vi "test Diff Configuration (Add Port).vi"(8 "error in":errorcluster, 11 "TestCase in":refnum<class "Refresh.lvclass">) -> (0 "error out":errorcluster, 3 "TestCase out":refnum<class "Refresh.lvclass">)   [LabVIEW 2020, in "Refresh.lvclass"]
uses:
  Refresh.lvclass
  System Explorer/Implementation/System Explorer/Refresh/MCL Row.ctl
  System Explorer/Implementation/System Explorer/Refresh/Change Type.ctl
  System Explorer/Implementation/System Explorer/Refresh/Symbols.ctl
  Shared/1553 Channel.ctl
  Shared/Address.ctl
  Shared/Message Definition.ctl
  Shared/Message Type.ctl
  Shared/Terminal Endpoint.ctl
  Shared/Parameter Definition.ctl
  <vilib>/addons/_JKI Toolkits/VI Tester/TestCase.llb/TestCase.lvclass
  System Explorer/Implementation/System Explorer/Refresh/Refresh.lvlib
  C:/Program Files (x86)/National Instruments/LabVIEW 2020/vi.lib/addons/_JKI Toolkits/VI Tester/TestCase.llb/TestCase.lvclass
panel:
  out "Multicolumn Listbox":i32(listbox)=-1
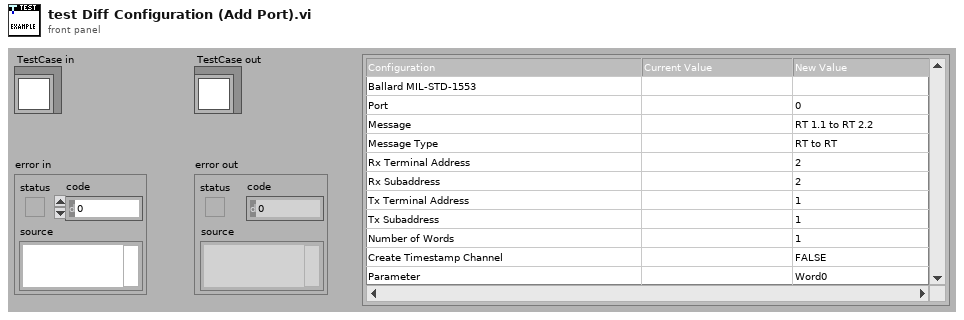
[diagram p1: front panel]
types:
  T1 = typedef "Message Definition.ctl" = cluster{"name":string, "message type":T2, "endpoint Tx":T3, "endpoint Rx":T3, "create timestamp channel":bool, "mode code":u16, "number of words":u16, "parameters":cluster{"name":string, "default value":dbl, "unit":string, "parameter definition":T5}[]}
  T2 = typedef "Message Type.ctl" = string
  T3 = typedef "Terminal Endpoint.ctl" = cluster{"terminal address":T4, "subaddress":T4}
  T4 = typedef "Address.ctl" = u16
  T5 = typedef "Parameter Definition.ctl" = cluster{"start index":i32, "size (bits)":i32, "encoding":enum16{"BNR", "BCD", "Discrete"}, "signed":bool, "multiplier":dbl, "offset":dbl}
  T6 = typedef "1553 Channel.ctl" = cluster{"HW channel":u16, "terminal addresses":T4[], "acyclic frame names":string[], "messages":T1[]}
  T7 = typedef "Ballard MIL-STD-1553 System Explorer.lvlib/Implementation.lvlib/Refresh.lvlib/MCL Row.ctl" = cluster{"change type":T8, "item symbol":T9, "item names":string[]}
  T8 = typedef "Ballard MIL-STD-1553 System Explorer.lvlib/Implementation.lvlib/Refresh.lvlib/Change Type.ctl" = enum16{"No change", "Modify", "Add", "Remove"}
  T9 = typedef "Ballard MIL-STD-1553 System Explorer.lvlib/Implementation.lvlib/Refresh.lvlib/Symbols.ctl" = enum16{"Blank", "MIL-STD-1553", "Port", "Remote Terminal", "Subaddress", "Bus Controller", "Acyclic Frame", "Mode Code", "Message", "Parameter", "Item"}
  T10 = typedef "imagedata.ctl" = cluster{"image type":i32, "image depth":i32, "image":u8[], "mask":u8[], "colors":u32[], "Rectangle":cluster{"left":i16, "top":i16, "right":i16, "bottom":i16}}
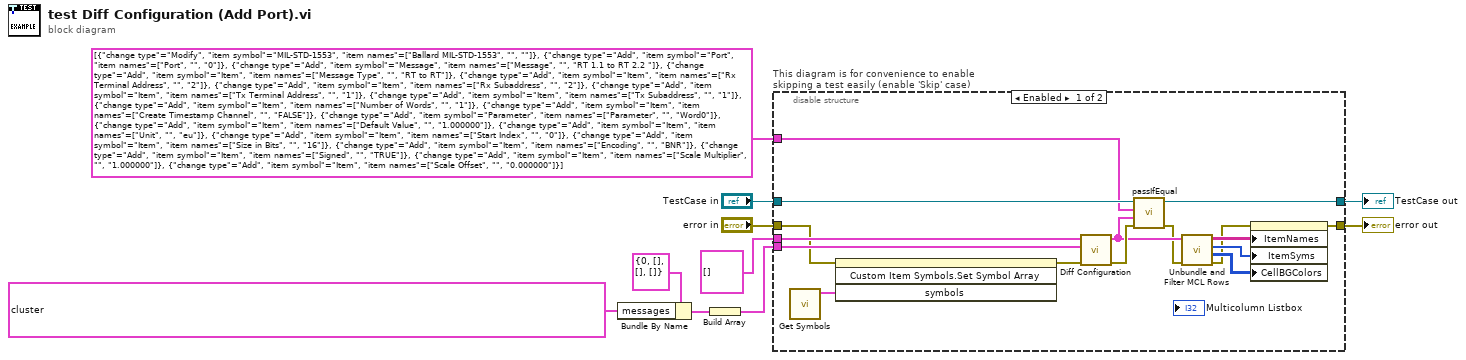
[diagram p0: block diagram]
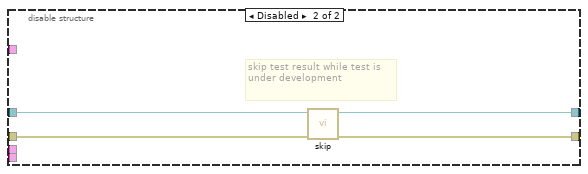
[diagram p2: hidden frame]
diagram:
  n1 = Bundle By Name(cluster=T6 {"HW channel"=0, "terminal addresses"=[], "acyclic frame names"=[], "messages"=[]} ("1553 channel"), "messages"=T1[] [{"name"="RT 1.1 to RT 2.2 ", "message type"="RT to RT", "endpoint Tx"={"terminal address"=1, "subaddress"=1}, "endpoint Rx"={"terminal address"=2, "subaddress"=2}, "create timestamp channel"=FALSE, "mode code"=0, "number of words"=1, "parameters"=[{"name"="Word0", "default value"=1.0, "unit"="eu", "parameter definition"={"start index"=0, "size (bits)"=16, "encoding"=enum."BNR", "signed"=TRUE, "multiplier"=1.0, "offset"=0.0}}]}]) -> (w1:T6)
  n2 = Build Array(w1) -> (w5:T6[])
  n3 = disable-structure "This diagram is for convenience to enable skipping a test easily (enable 'Skip' case)" shown="Enabled" {
    disable-tunnel: "TestCase in" -> [w26 w30]
    disable-tunnel: [w25 w28] -> w7
    disable-tunnel: [w14 w29] -> w9
    disable-tunnel: "error in" -> [w12 w27]
    disable-tunnel: T6[] [] -> [w24 _]
    disable-tunnel: w5 -> [w23 _]
    disable-tunnel: T7[] [{"change type"=enum."Modify", "item symbol"=enum."MIL-STD-1553", "item names"=["Ballard MIL-STD-1553", "", ""]}, {"change type"=enum."Add", "item symbol"=enum."Port", "item names"=["Port", "", "0"]}, {"change type"=enum."Add", "item symbol"=enum."Message", "item names"=["Message", "", "RT 1.1 to RT 2.2 "]}, {"change type"=enum."Add", "item symbol"=enum."Item", "item names"=["Message Type", "", "RT to RT"]}, {"change type"=enum."Add", "item symbol"=enum."Item", "item names"=["Rx Terminal Address", "", "2"]}, {"change type"=enum."Add", "item symbol"=enum."Item", "item names"=["Rx Subaddress", "", "2"]}, {"change type"=enum."Add", "item symbol"=enum."Item", "item names"=["Tx Terminal Address", "", "1"]}, {"change type"=enum."Add", "item symbol"=enum."Item", "item names"=["Tx Subaddress", "", "1"]}, {"change type"=enum."Add", "item symbol"=enum."Item", "item names"=["Number of Words", "", "1"]}, {"change type"=enum."Add", "item symbol"=enum."Item", "item names"=["Create Timestamp Channel", "", "FALSE"]}, {"change type"=enum."Add", "item symbol"=enum."Parameter", "item names"=["Parameter", "", "Word0"]}, {"change type"=enum."Add", "item symbol"=enum."Item", "item names"=["Default Value", "", "1.000000"]}, {"change type"=enum."Add", "item symbol"=enum."Item", "item names"=["Unit", "", "eu"]}, {"change type"=enum."Add", "item symbol"=enum."Item", "item names"=["Start Index", "", "0"]}, {"change type"=enum."Add", "item symbol"=enum."Item", "item names"=["Size in Bits", "", "16"]}, {"change type"=enum."Add", "item symbol"=enum."Item", "item names"=["Encoding", "", "BNR"]}, {"change type"=enum."Add", "item symbol"=enum."Item", "item names"=["Signed", "", "TRUE"]}, {"change type"=enum."Add", "item symbol"=enum."Item", "item names"=["Scale Multiplier", "", "1.000000"]}, {"change type"=enum."Add", "item symbol"=enum."Item", "item names"=["Scale Offset", "", "0.000000"]}] ("configuration diff") -> [w22 _]
    frame Enabled {
      n4 = call "Get Symbols.vi"() -> ("MIL-STD-1553 symbols"=w13:T10[])  [unwired: 11 in]
      n5 = invoke on="Multicolumn Listbox" class="MCListbox (strict)" method="Custom Item Symbols.Set Symbol Array"(error in=w12, "symbols"=w13) -> (error out=w11:errorcluster)  [unwired: 2 in, 3 out]
      n6 = call "Diff Configuration.vi"("error in"=w11, "configuration new"=w23, "configuration old"=w24) -> ("error out"=w21:errorcluster, "configuration diff"=w20:T7[])  [unwired: 7 in]
      n7 = call-dynamic "passIfEqual.vi"("error in (no error)"=w21, "y"=w20, "x"=w22, "TestCase in"=w26) -> ("error out"=w16:errorcluster, "TestCase out"=w25:refnum<class "Refresh.lvclass">)  [unwired: 6 in]
      n8 = call "Unbundle and Filter MCL Rows.vi"("error in"=w16, "refresh items"=w20) -> ("error out"=w15:errorcluster, "background colors"=w19:u32[][], "item symbols"=w18:T9[], "item names"=w17:string[][])  [unwired: 6 in]
      n9 = property on="Multicolumn Listbox" class="MCListbox (strict)"(error in=w15, "ItemNames"=w17, "ItemSyms"=w18, "CellBGColors"=w19) -> (error out=w14:errorcluster)  [unwired: 1 in, 1 out]
    }
    frame Disabled {
      # "skip test result while test is under development"
      n10 = call <vilib>:"skip.vi"("error in (no error)"=w27, "TestCase in"=w30) -> ("error out"=w29:errorcluster, "TestCase out"=w28:refnum<class "Refresh.lvclass">)  [unwired: 8 in]
    }
  }
  "error out" <- w9
  "TestCase out" <- w7
